vi "test-TimeInterpDouble-Test1.vi"() -> (3 "All tests passed":bool)   [LabVIEW 2019]
uses:
  <vilib>/Rock Robotics/WPI/ThirdParty/JAS_Junk/TrajLib/Trajectory_Library.lvlib
  <vilib>/Rock Robotics/WPI/ThirdParty/JAS_Junk/TrajLib/TIME_INTERPOLATABLE_DOUBLE.ctl
panel:
  out "out TimeInterpDouble":T1
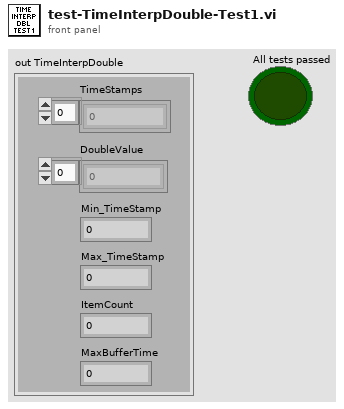
[diagram p1: front panel]
types:
  T1 = typedef "Trajectory_Library.lvlib/TIME_INTERPOLATABLE_DOUBLE.ctl" = cluster{"TimeStamps":dbl[], "DoubleValue":dbl[], "Min_TimeStamp":dbl, "Max_TimeStamp":dbl, "ItemCount":i32, "MaxBufferTime":dbl}
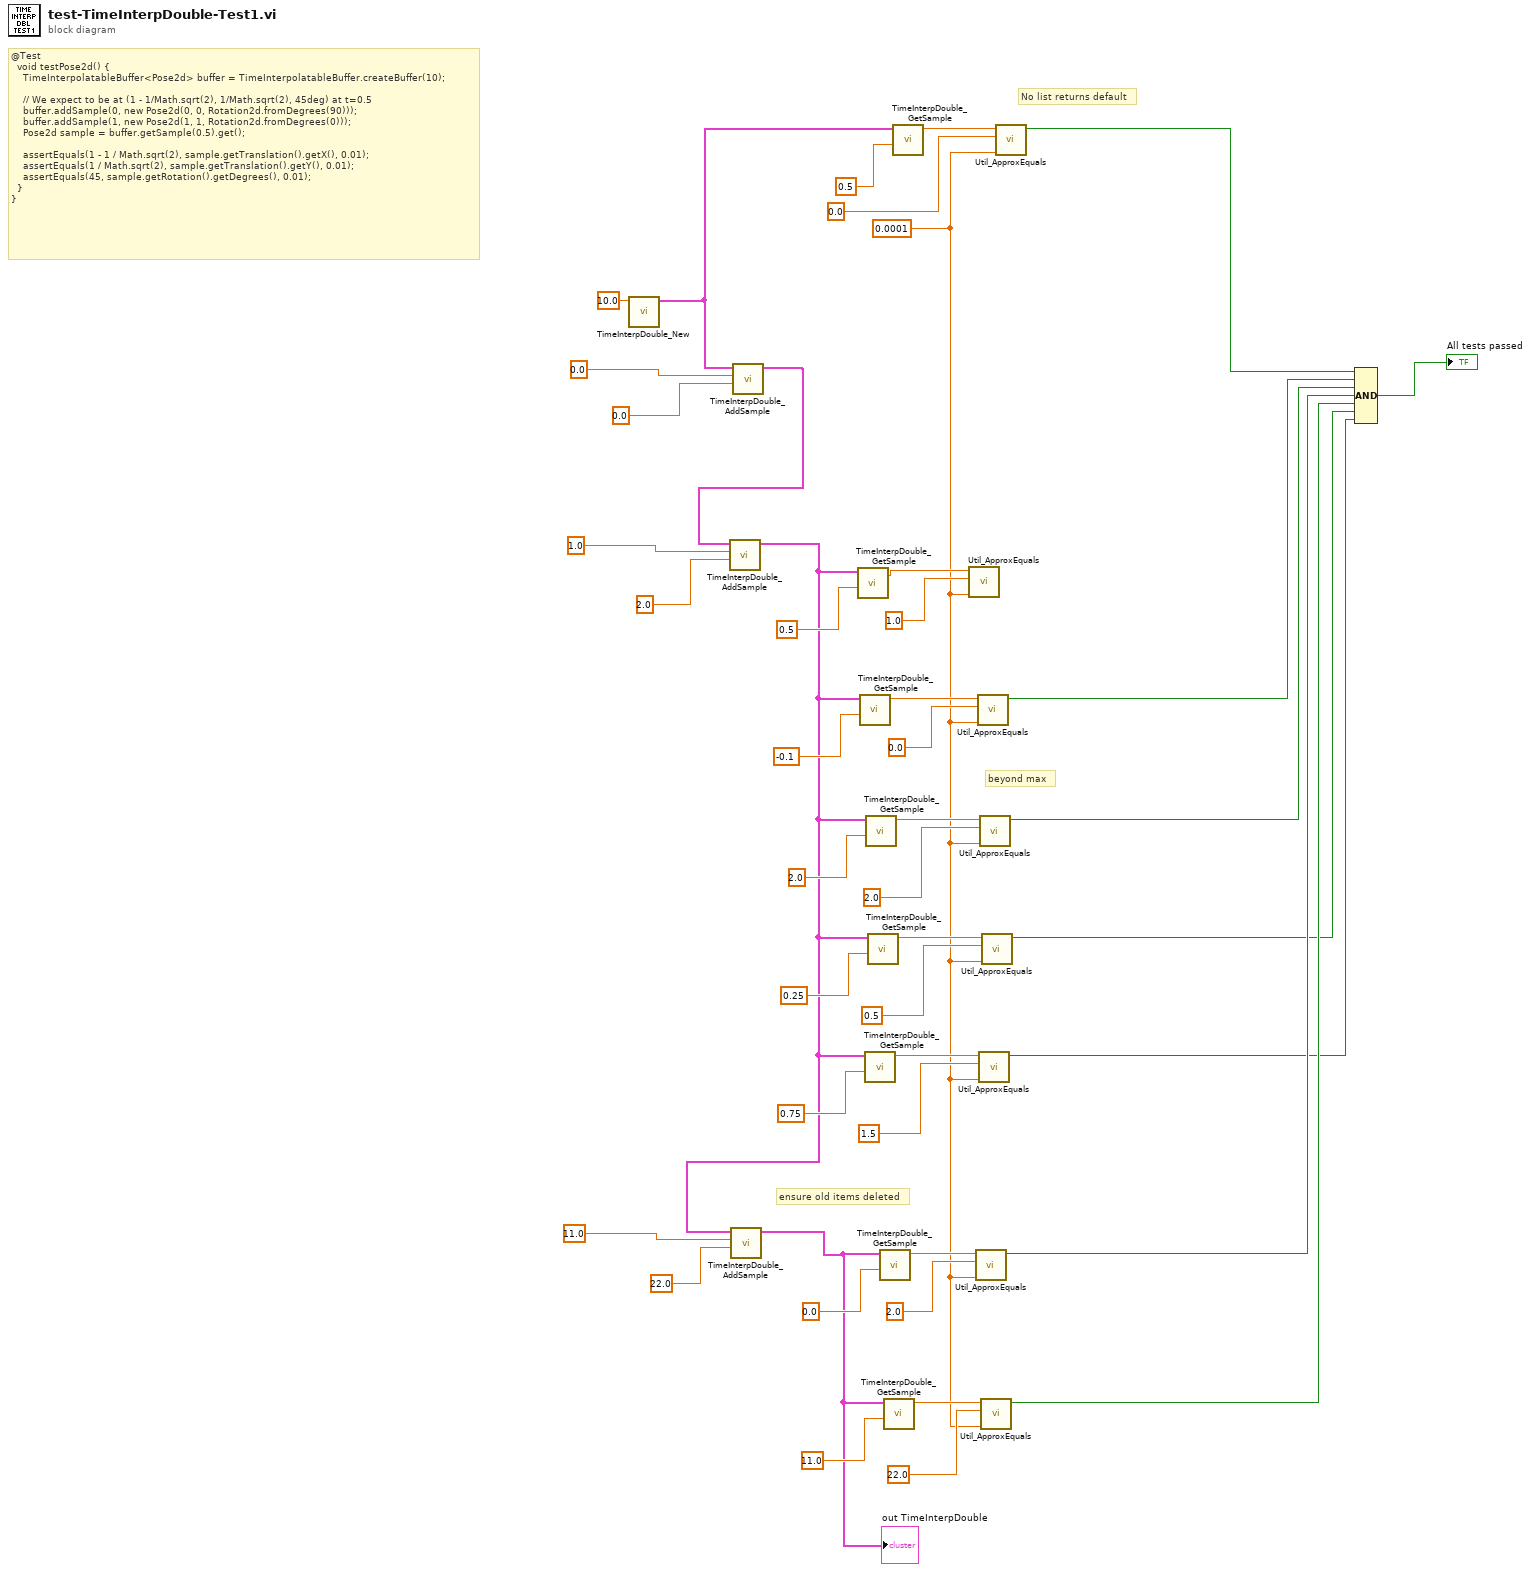
[diagram p0: block diagram]
diagram:
  w4 = 0.0001 ("Tolerance")
  # "beyond max"
  # "ensure old items deleted"
  # "No list returns default"
  # "@Test\n  void testPose2d() {\n    TimeInterpolatableBuffer<Pose2d> buffer = TimeInterpolatableBuffer.createBuffer(10);\n\n    // We expect to be at (1 - 1/Math.sqrt(2), 1/Math.sqrt(2), 45deg) at t=0.5\n    buffer.addSample(0, new Pose2d(0, 0, Rotation2d.fromDegrees(90)));\n    buffer.addSample(1, new Pose2d(1, 1, Rotation2d.fromDegrees(0)));\n    Pose2d sample = buffer.getSample(0.5).get();\n\n    assertEquals(1 - 1 / Math.sqrt(2), sample.getTranslation().getX(), 0.01);\n    assertEquals(1 / Math.sqrt(2), sample.getTranslation().getY(), 0.01);\n    assertEquals(45, sample.getRotation().getDegrees(), 0.01);\n  }\n}"
  n1 = call <vilib>:"TimeInterpDouble_New.vi"("MaxTime"=10.0) -> ("TimeInterpDouble"=w36:T1)  [unwired: 10 in]
  n2 = call <vilib>:"TimeInterpDouble_AddSample.vi"("Value"=0.0, "TimeStamp"=0.0, "in TimeInterpDouble"=w36) -> ("out TimeInterpDouble"=w38:T1)  [unwired: 7 in, 1 out]
  n3 = call <vilib>:"TimeInterpDouble_AddSample.vi"("Value"=2.0, "TimeStamp"=1.0, "in TimeInterpDouble"=w38) -> ("out TimeInterpDouble"=w1:T1)  [unwired: 7 in, 1 out]
  n4 = call <vilib>:"TimeInterpDouble_AddSample.vi"("Value"=22.0, "TimeStamp"=11.0, "in TimeInterpDouble"=w1) -> ("out TimeInterpDouble"=w24:T1)  [unwired: 7 in, 1 out]
  "out TimeInterpDouble" <- w24
  n5 = call <vilib>:"TimeInterpDouble_GetSample.vi"("TimeStamp"=0.5, "TimeInterpDouble"=w1) -> ("OutputDouble"=w21:dbl)  [unwired: 9 in]
  n6 = call <vilib>:"TimeInterpDouble_GetSample.vi"("TimeStamp"=-0.1, "TimeInterpDouble"=w1) -> ("OutputDouble"=w34:dbl)  [unwired: 9 in]
  n7 = call <vilib>:"TimeInterpDouble_GetSample.vi"("TimeStamp"=0.75, "TimeInterpDouble"=w1) -> ("OutputDouble"=w6:dbl)  [unwired: 9 in]
  n8 = call <vilib>:"TimeInterpDouble_GetSample.vi"("TimeStamp"=2.0, "TimeInterpDouble"=w1) -> ("OutputDouble"=w32:dbl)  [unwired: 9 in]
  n9 = call <vilib>:"TimeInterpDouble_GetSample.vi"("TimeStamp"=0.25, "TimeInterpDouble"=w1) -> ("OutputDouble"=w9:dbl)  [unwired: 9 in]
  n10 = call <vilib>:"TimeInterpDouble_GetSample.vi"("TimeStamp"=0.0, "TimeInterpDouble"=w24) -> ("OutputDouble"=w27:dbl)  [unwired: 9 in]
  n11 = call <vilib>:"TimeInterpDouble_GetSample.vi"("TimeStamp"=11.0, "TimeInterpDouble"=w24) -> ("OutputDouble"=w25:dbl)  [unwired: 9 in]
  n12 = call <vilib>:"TimeInterpDouble_GetSample.vi"("TimeStamp"=0.5, "TimeInterpDouble"=w36) -> ("OutputDouble"=w37:dbl)  [unwired: 9 in]
  n13 = call <vilib>:"Util_ApproxEquals.vi"("Tolerance"=w4, "Value 2"=1.0, "Value 1"=w21) -> ()  [unwired: 8 in, 1 out]
  n14 = call <vilib>:"Util_ApproxEquals.vi"("Tolerance"=w4, "Value 2"=2.0, "Value 1"=w27) -> ("ApproxEquals"=w23:bool)  [unwired: 8 in]
  n15 = call <vilib>:"Util_ApproxEquals.vi"("Tolerance"=w4, "Value 2"=0.0, "Value 1"=w34) -> ("ApproxEquals"=w31:bool)  [unwired: 8 in]
  n16 = call <vilib>:"Util_ApproxEquals.vi"("Tolerance"=w4, "Value 2"=1.5, "Value 1"=w6) -> ("ApproxEquals"=w2:bool)  [unwired: 8 in]
  n17 = call <vilib>:"Util_ApproxEquals.vi"("Tolerance"=w4, "Value 2"=2.0, "Value 1"=w32) -> ("ApproxEquals"=w30:bool)  [unwired: 8 in]
  n18 = call <vilib>:"Util_ApproxEquals.vi"("Tolerance"=w4, "Value 2"=22.0, "Value 1"=w25) -> ("ApproxEquals"=w22:bool)  [unwired: 8 in]
  n19 = call <vilib>:"Util_ApproxEquals.vi"("Tolerance"=w4, "Value 2"=0.5, "Value 1"=w9) -> ("ApproxEquals"=w3:bool)  [unwired: 8 in]
  n20 = call <vilib>:"Util_ApproxEquals.vi"("Tolerance"=w4, "Value 2"=0.0, "Value 1"=w37) -> ("ApproxEquals"=w15:bool)  [unwired: 8 in]
  n21 = Compound Arithmetic op=AND(w15, w31, w30, w23, w22, w3, w2) -> (→"All tests passed":bool)
